vi "ArrayWaveforms.vi"(8 "error in (no error)":errorcluster, 9 "Probe Name":string, 10 "open Probe":bool=TRUE, 11 "Probe":waveform(dbl)[](array[waveform])) -> (0 "error out":errorcluster)   [LabVIEW 2010]
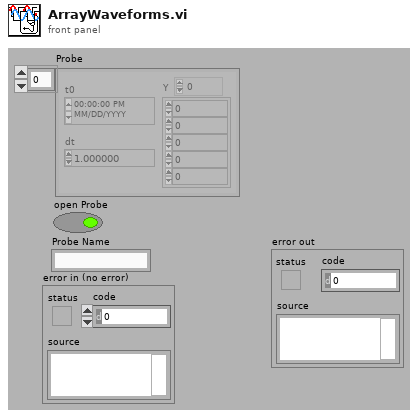
[diagram p1: front panel]
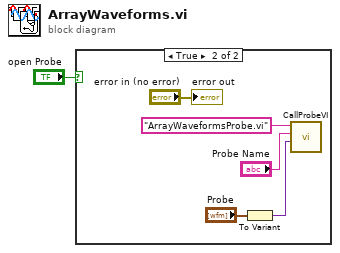
[diagram p0: block diagram]
diagram:
  n1 = case shown="True" "open Probe" {
    frame False {
    }
    frame True {
      n2 = To Variant(anything="Probe") -> (Variant=w4:variant)
      n3 = call "CallProbeVI.vi"("Data"=w4, "Probe Name"="Probe Name", "Probe VI Name"="ArrayWaveformsProbe.vi" ("name or relative path")) -> ()  [unwired: 9 in]
      "error out" <- "error in (no error)"
    }
  }
